vi "PIFOCS Controller.vi"() -> ()   [LabVIEW 2015]
uses:
  PiFOC State.ctl
  GCS_LabVIEW/PiFOC.lvlib
panel:
  out "State":T1
  out "Waveform Chart":dbl(graph)
  out "error out":errorcluster
  out "Identification":string
  in  "stop":bool
  out "Position":dbl
  in  "Piezo Go To /um":dbl(slide) scale=0.0..100.0
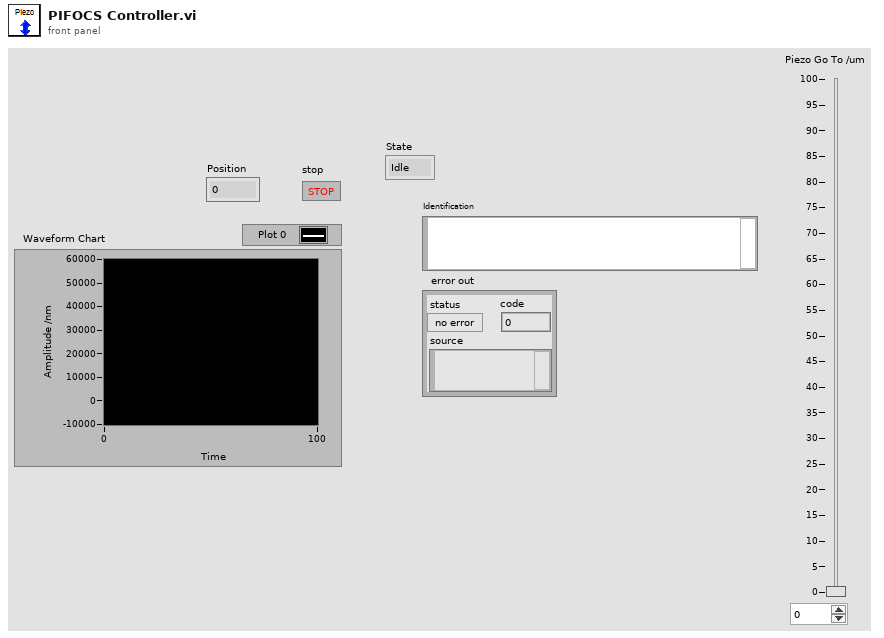
[diagram p1: front panel]
types:
  T1 = typedef "PiFOC State.ctl" = enum16{"Idle", "GoTo", "getPosition"}
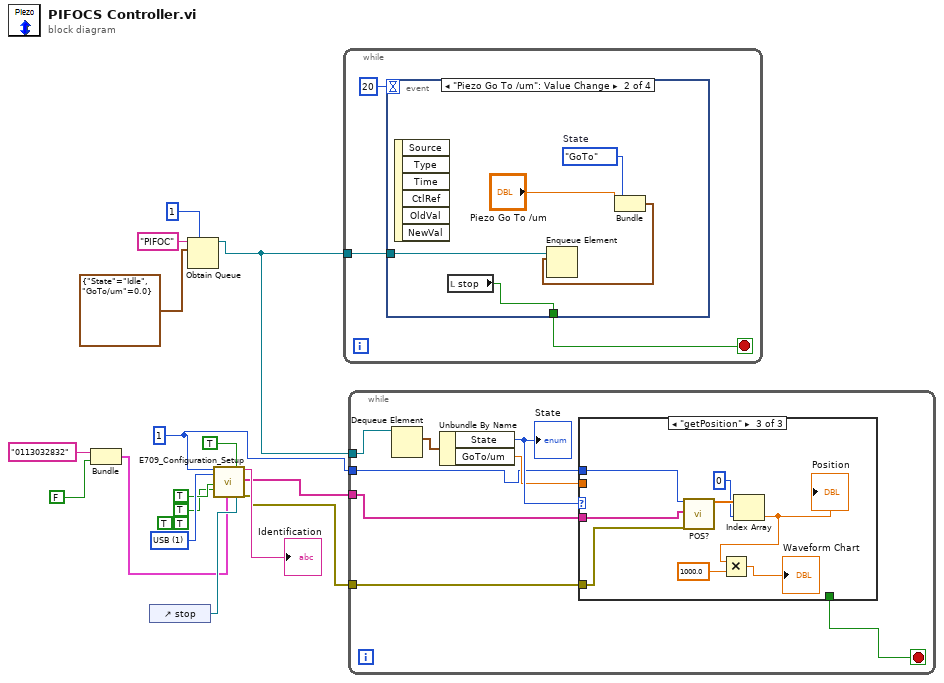
[diagram p0: block diagram]
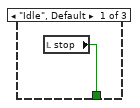
[diagram p2: hidden frame]
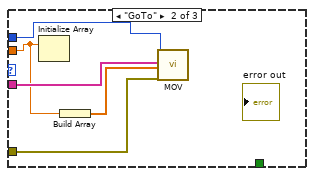
[diagram p3: hidden frame]
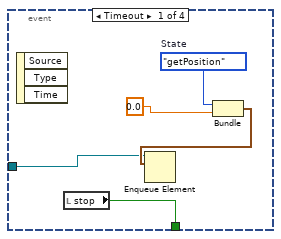
[diagram p4: hidden frame]
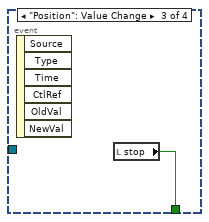
[diagram p5: hidden frame]
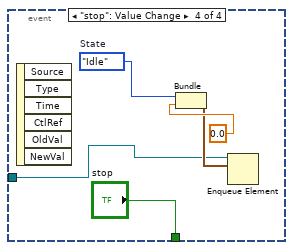
[diagram p6: hidden frame]
diagram:
  w6 = 1 ("System no.")
  (unwired) TRUE ("Connected?")
  (unwired) TRUE ("Connected?")
  w13 = u16 1 items=["RS232", "USB"] ("Interface")
  n1 = Bundle("Serial Number"="0113032832", FALSE) -> (w2:cluster{"Serial Number":string, bool})  [unwired: 1 in]
  n2 = control-ref of="stop"() -> (w9:refnum<vi>)
  n3 = Obtain Queue(max queue size (-1, unlimited)=1, name (unnamed)="PIFOC", element data type=cluster{"State":T1, "GoTo/um":dbl} {"State"=enum."Idle", "GoTo/um"=0.0} ("input cluster")) -> (queue out=w14:refnum<queue>)  [unwired: 2 in, 2 out]
  n4 = call "E709_Configuration_Setup.vi"("System no."=w6, "Interface"=w13, "Change servo status to ON?"=TRUE, "Perform autozero?"=TRUE, "USB settings"=w2, "Move to middle?"=TRUE, "Stop refnum"=w9) -> ("Identification"=→"Identification":string, "Conn. \nAxis"=w7:string[], "error out"=w5:errorcluster)  [unwired: 7 in, 3 out]
  n5 = while {
    tunnel: w14 -> [w19]
    stop <- w18 stop-if-true
    n6 = event shown="[1] \"Piezo Go To /um\": Value Change" {
      selector: _ -> [_ _ _ _]
      dyn-events: _ -> [_ _ _ _]
      timeout: 20 -> [_ _ _ _]
      tunnel: w19 -> [w22 w29 _ w31]
      tunnel: [w20 w25 w30 "stop"] -> w18
      event Timeout {
        w24 = PiFOC_State."getPosition"  # State
        n7 = event-data() -> ()  [unwired: 1 in, 3 out]
        n8 = local read "stop"() -> (w20:bool)
        n9 = Bundle("State"=w24, 0.0) -> (w23:cluster{"State":T1, dbl})  [unwired: 1 in]
        n10 = Enqueue Element(queue=w22, element=w23) -> ()  [unwired: 2 in, 3 out]
      }
      event "Piezo Go To /um": Value Change {
        w27 = PiFOC_State."GoTo"  # State
        n11 = event-data() -> ()  [unwired: 1 in, 6 out]
        n12 = local read "stop"() -> (w25:bool)
        n13 = Bundle("State"=w27, "Piezo Go To /um"="Piezo Go To /um") -> (w26:cluster{"State":T1, "Piezo Go To /um":dbl})  [unwired: 1 in]
        n14 = Enqueue Element(queue=w29, element=w26) -> ()  [unwired: 2 in, 3 out]
      }
      event "Position": Value Change {
        n15 = event-data() -> ()  [unwired: 1 in, 6 out]
        n16 = local read "stop"() -> (w30:bool)
      }
      event "stop": Value Change {
        w33 = PiFOC_State."Idle"  # State
        n17 = event-data() -> ()  [unwired: 1 in, 6 out]
        n18 = Bundle("State"=w33, 0.0) -> (w32:cluster{"State":T1, dbl})  [unwired: 1 in]
        n19 = Enqueue Element(queue=w31, element=w32) -> ()  [unwired: 2 in, 3 out]
      }
    }
  }
  n20 = while {
    tunnel: w14 -> [w43]
    tunnel: w7 -> [w39]
    tunnel: w6 -> [w38]
    tunnel: w5 -> [w37]
    stop <- w36 stop-if-true
    n21 = Dequeue Element(queue=w43) -> (element=w42:cluster{"State":T1, "GoTo/um":dbl})  [unwired: 2 in, 3 out]
    n22 = Unbundle By Name(w42) -> ("State"=w41:T1, "GoTo/um"=w40:dbl)
    "State" <- w41
    n23 = case shown="\"getPosition\"" w41 {
      tunnel: w40 -> [_ w46 _]
      tunnel: w39 -> [_ w49 w54]
      tunnel: w38 -> [_ w47 w55]
      tunnel: w37 -> [_ w48 w53]
      tunnel: [w44 _ _] -> w36
      frame "Idle", Default {
        n24 = local read "stop"() -> (w44:bool)
      }
      frame "GoTo" {
        n25 = Initialize Array(w46) -> ()  [unwired: 1 in, 1 out]
        n26 = Build Array(w46) -> (w45:dbl[])
        n27 = call "MOV.vi"("System no."=w47, "Axes to move"=w49, "Position values"=w45, "error in"=w48) -> ()  [unwired: 15 in, 1 out]
      }
      frame "getPosition" {
        n28 = call "POS?.vi"("System no."=w55, "Axes to query"=w54, "error in"=w53) -> ("Position"=w57:dbl[])  [unwired: 15 in, 1 out]
        n29 = Index Array(array=w57, index=0) -> (element=w52:dbl)
        "Position" <- w52
        n30 = Multiply(x=w52, y=1000.0) -> (x*y=→"Waveform Chart":dbl)
      }
    }
  }
